vi "(SubVI)Waveform Editor_Update Sampling Rate Value.vi"(7 "Action":T1=enum."Update", 8 "error in (no error)":errorcluster caption="에러 입력(에러 없음)", 10 "Sampling Rate Ref":refnum<vi>, 11 "Value":u8) -> (0 "error out":errorcluster caption="에러 출력")   [LabVIEW 2020]
uses:
  Controls/(Ctrl)Waveform Editor_Update Sampling Rate Value.ctl
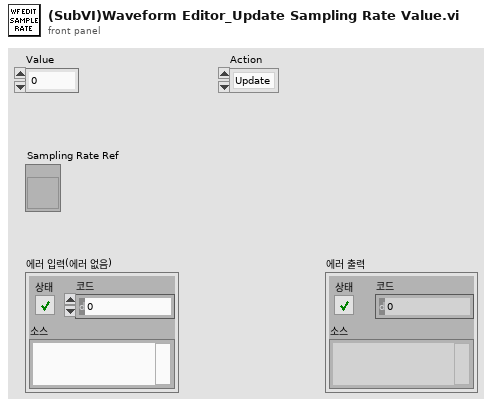
[diagram p1: front panel]
types:
  T1 = typedef "(Ctrl)Waveform Editor_Update Sampling Rate Value.ctl" = enum16{"Init", "Update"}
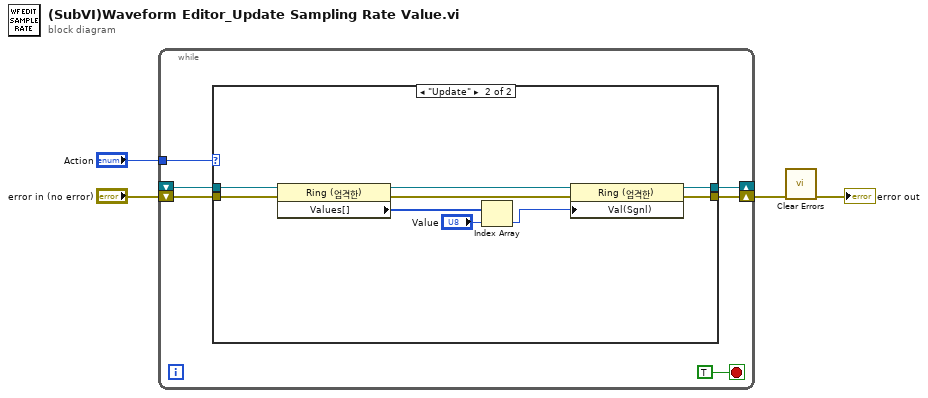
[diagram p0: block diagram]
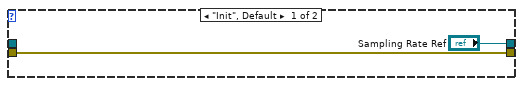
[diagram p2: hidden frame]
diagram:
  n1 = while {
    tunnel: "Action" -> [w9]
    shift-right: [w8] -> _
    shift-left: _ -> [w5]
    shift-right: [w7] -> w3
    shift-left: "error in (no error)" -> [w6]
    stop <- TRUE stop-if-true
    n2 = case shown="\"Update\"" w9 {
      tunnel: ["Sampling Rate Ref" w16] -> w8
      tunnel: [w12 w15] -> w7
      tunnel: w6 -> [w12 w13]
      tunnel: w5 -> [_ w14]
      frame "Init", Default {
      }
      frame "Update" {
        n3 = property class="Ring (엄격한)"(reference=w14, error in=w13) -> (reference out=w19:refnum<vi>, error out=w18:errorcluster, "Values[]"=w21:u32[])
        n4 = Index Array(array=w21, index="Value") -> (element=w17:u32)
        n5 = property class="Ring (엄격한)"(reference=w19, error in=w18, "Val(Sgnl)"=w17) -> (reference out=w16:refnum<vi>, error out=w15:errorcluster)
      }
    }
  }
  n6 = call <vilib>:"Clear Errors.vi"("error in (no error)"=w3) -> ("error out"=→"error out":errorcluster)  [unwired: 5 in, 1 out]
